vi "vi_reference_read.vi"(8 "error in (no error)":errorcluster, 11 "interface in":refnum<class "interface.lvclass">) -> (0 "error out":errorcluster, 2 "vi_reference":T1, 3 "interface out":refnum<class "interface.lvclass">)   [LabVIEW 2015, in "functional.lvlib" / "interface.lvclass"]
uses:
  interface.lvclass
  _controls/vi_reference.ctl
  interface.lvclass/interface.ctl
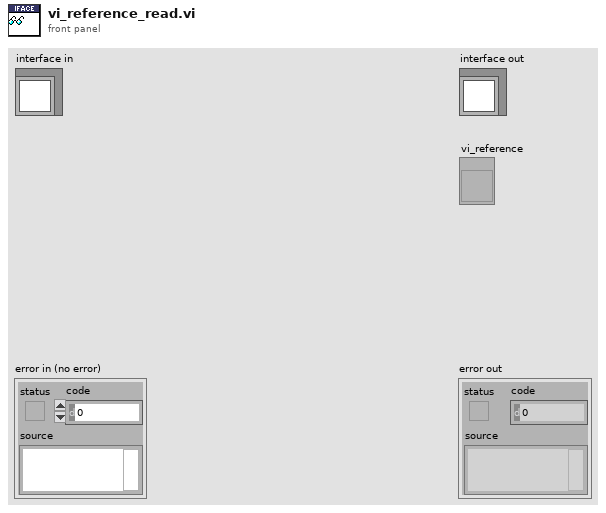
[diagram p1: front panel]
types:
  T1 = typedef "functional.lvlib/interface.lvclass/vi_reference.ctl" = refnum<vi>
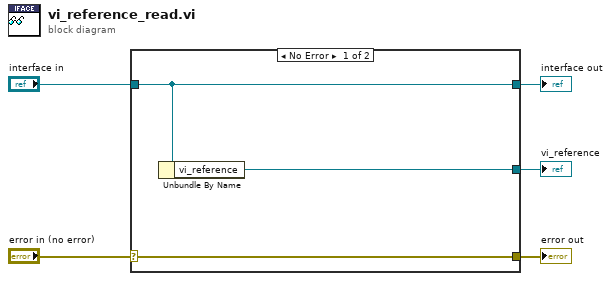
[diagram p0: block diagram]
diagram:
  n1 = case shown="No Error" "error in (no error)" {
    selector: "error in (no error)" -> [w8 w9]
    tunnel: [w8 w9] -> w4
    tunnel: [w7 w10] -> w2
    tunnel: "interface in" -> [w7 w10]
    tunnel: [w6 _] -> w1
    frame No Error {
      n2 = Unbundle By Name(w7) -> ("vi_reference"=w6:T1)
    }
    frame Error {
    }
  }
  "error out" <- w4
  "interface out" <- w2
  "vi_reference" <- w1
